vi "S101_BC79.vi"(0 "Loop Meas":T5, 1 "Redudancy 1 Meas":T4, 2 "Redudancy 2 Meas":T3, 3 "Redudancy 3 Meas":T2, 4 "Redudancy 4 Meas":T1, 5 "error in (no error)":errorcluster) -> (16 "ACT D-Comp":dbl)   [LabVIEW 2022 SP3, in "SI101_AverageReactorCoolantTemperature.lvclass"]
uses:
  SI101_AverageReactorCoolantTemperature.lvclass
  SI101_AverageReactorCoolantTemperature.lvclass/SI101_AverageReactorCoolantTemperature.ctl
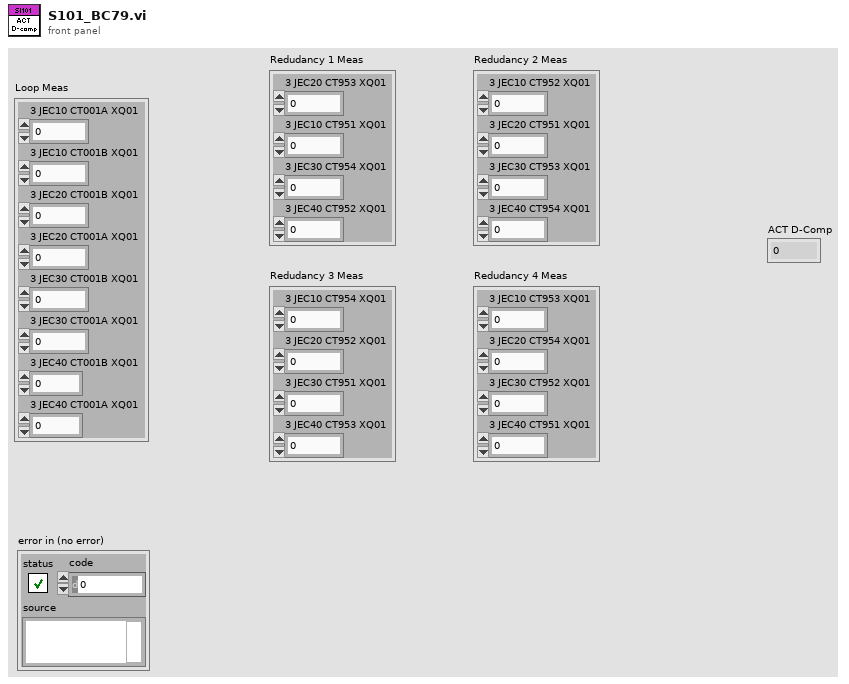
[diagram p1: front panel]
types:
  T1 = cluster{"3 JEC10 CT953 XQ01":dbl, "3 JEC20 CT954 XQ01":dbl, "3 JEC30 CT952 XQ01":dbl, "3 JEC40 CT951 XQ01":dbl}
  T2 = cluster{"3 JEC10 CT954 XQ01":dbl, "3 JEC20 CT952 XQ01":dbl, "3 JEC30 CT951 XQ01":dbl, "3 JEC40 CT953 XQ01":dbl}
  T3 = cluster{"3 JEC10 CT952 XQ01":dbl, "3 JEC20 CT951 XQ01":dbl, "3 JEC30 CT953 XQ01":dbl, "3 JEC40 CT954 XQ01":dbl}
  T4 = cluster{"3 JEC20 CT953 XQ01":dbl, "3 JEC10 CT951 XQ01":dbl, "3 JEC30 CT954 XQ01":dbl, "3 JEC40 CT952 XQ01":dbl}
  T5 = cluster{"3 JEC10 CT001A XQ01":dbl, "3 JEC10 CT001B XQ01":dbl, "3 JEC20 CT001B XQ01":dbl, "3 JEC20 CT001A XQ01":dbl, "3 JEC30 CT001B XQ01":dbl, "3 JEC30 CT001A XQ01":dbl, "3 JEC40 CT001B XQ01":dbl, "3 JEC40 CT001A XQ01":dbl}
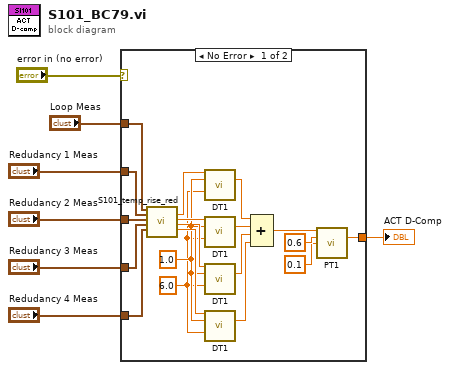
[diagram p0: block diagram]
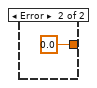
[diagram p2: hidden frame]
diagram:
  n1 = case shown="No Error" "error in (no error)" {
    tunnel: "Loop Meas" -> [w26 _]
    tunnel: "Redudancy 1 Meas" -> [w25 _]
    tunnel: "Redudancy 2 Meas" -> [w24 _]
    tunnel: "Redudancy 3 Meas" -> [w23 _]
    tunnel: "Redudancy 4 Meas" -> [w22 _]
    tunnel: [w8 0.0 ("output y(k)")] -> w1
    frame No Error {
      w16 = 6.0 ("T1")
      w17 = 1.0 ("G")
      n2 = call "S101_temp_rise_red.vi"("Loop Meas"=w26, "Redudancy 1 Meas"=w25, "Redudancy 2 Meas"=w24, "Redudancy 3 Meas"=w23, "Redudancy 4 Meas"=w22) -> ("ACT Loop 1"=w21:dbl, "ACT Loop 2"=w20:dbl, "ACT loop 3"=w19:dbl, "ACT loop 4"=w18:dbl)  [unwired: 11 in]
      n3 = call "DT1.vi"("input u(k)"=w21, "G"=w17, "T1"=w16) -> ("output y(k)"=w15:dbl)  [unwired: 11 in, 1 out]
      n4 = call "DT1.vi"("input u(k)"=w20, "G"=w17, "T1"=w16) -> ("output y(k)"=w14:dbl)  [unwired: 11 in, 1 out]
      n5 = call "DT1.vi"("input u(k)"=w19, "G"=w17, "T1"=w16) -> ("output y(k)"=w13:dbl)  [unwired: 11 in, 1 out]
      n6 = call "DT1.vi"("input u(k)"=w18, "G"=w17, "T1"=w16) -> ("output y(k)"=w12:dbl)  [unwired: 11 in, 1 out]
      n7 = Compound Arithmetic op=ADD(w15, w14, w13, w12) -> (w11:dbl)
      n8 = call "PT1.vi"("input u(k)"=w11, "G"=0.6, "T1"=0.1) -> ("output y(k)"=w8:dbl)  [unwired: 11 in, 1 out]
    }
    frame Error {
    }
  }
  "ACT D-Comp" <- w1
